vi "enterIPAddress.vi"(0 "IP Address":string="10.0.0.55") -> (1 "IP Address Out":string, 2 "Was Canceled":bool)   [LabVIEW 2019, in "h.Library.lvlib"]
uses:
  h.Library.lvlib
panel:
  in  "Cancel Button":bool
  in  "OK Button":bool
  # "Specify the IP Address for the instrument\nthat you are trying to connect to."
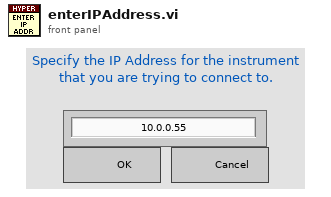
[diagram p1: front panel]
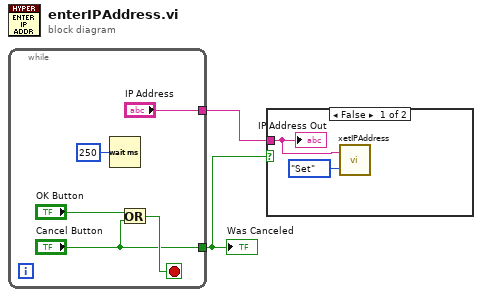
[diagram p0: block diagram]
diagram:
  n1 = while {
    tunnel: ["IP Address"] -> w1
    tunnel: ["Cancel Button"] -> w2
    stop <- w6 stop-if-true
    n2 = Wait (ms)(milliseconds to wait=u32 250) -> ()  [unwired: 1 out]
    n3 = Or(x="OK Button", y="Cancel Button") -> (x .or. y?=w6:bool)
  }
  "Was Canceled" <- w2
  n4 = case shown="False" w2 {
    tunnel: w1 -> [w8 _]
    frame False {
      n5 = call "xetIPAddress.vi"("Get/Set"=enum16{"Get", "Set"}."Set", "IP Address In"=w8) -> ()  [unwired: 1 out]
      "IP Address Out" <- w8
    }
    frame True {
    }
  }
